vi "daqio_get_dashboard.vi"(8 "error in":errorcluster, 11 "daq.io type in":T3={"daq.io ref"=refnum, "daq.io API Base"="http://dashboard.daq.io/api/v1", "Device Key"="", "Account ID"="", "online"=TRUE, "SSL"=TRUE, "buffer"=TRUE}) -> (0 "error out":errorcluster, 2 "dashboards":T1, 3 "daq.io type out":T3={"daq.io ref"=refnum, "daq.io API Base"="http://dashboard.daq.io/api/v1", "Device Key"="", "Account ID"="", "online"=TRUE, "SSL"=TRUE, "buffer"=TRUE})   [LabVIEW 2013, in "daqio minimal.lvlib"]
doc: "This VI creates a new default dashboard for a specific account and makes it the new default dashboard for the current device."
uses:
  daqio minimal.lvlib
  _typedefs/daqio-Type.ctl
  <vilib>/httpClient/ClientHandle.ctl
  _typedefs/daqio-Device-Just-Dashboards.ctl
  _typedefs/daqio-Device-Dashboards.ctl
  <vilib>/Easy HTTP Client/Easy HTTP.lvlib
  <vilib>/httpClient/LabVIEWHTTPClient.lvlib
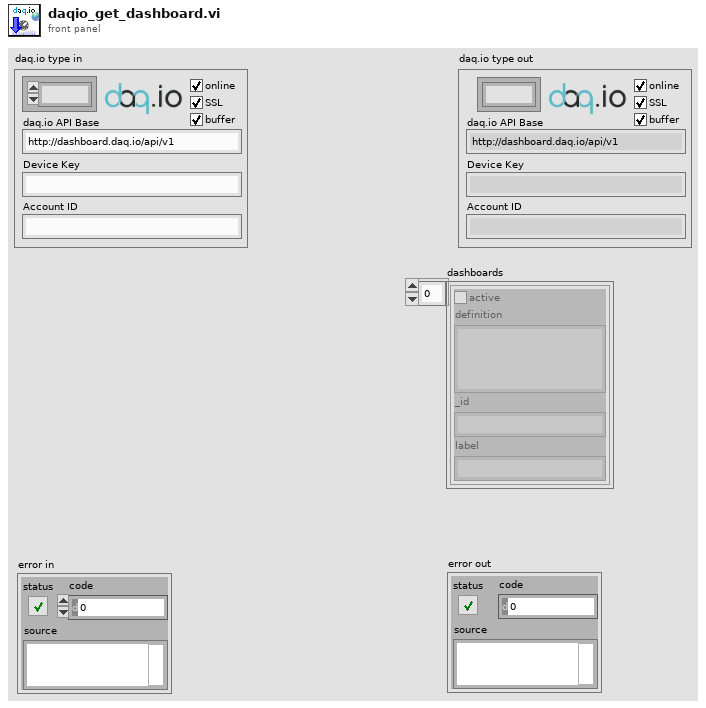
[diagram p1: front panel]
types:
  T1 = typedef "daqio minimal.lvlib/daqio-Device-Just-Dashboards.ctl" = T2[]
  T2 = typedef "daqio minimal.lvlib/daqio-Device-Dashboards.ctl" = cluster{"active":bool, "definition":string, "_id":string, "label":string}
  T3 = typedef "daqio minimal.lvlib/daqio-Type.ctl" = cluster{"daq.io ref":T4, "daq.io API Base":string, "Device Key":string, "Account ID":string, "online":bool, "SSL":bool, "buffer":bool}
  T4 = typedef "LabVIEWHTTPClient.lvlib/ClientHandle.ctl" = refnum<k1>
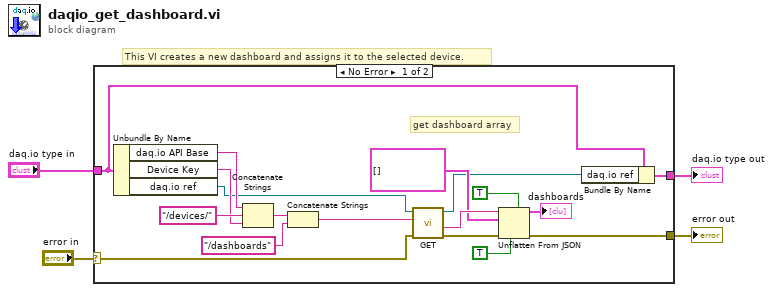
[diagram p0: block diagram]
diagram:
  # "This VI creates a new dashboard and assigns it to the selected device."
  n1 = case shown="No Error" "error in" {
    selector: "error in" -> [w8 w23]
    tunnel: "daq.io type in" -> [w10 w24]
    tunnel: [w21 w24] -> w3
    tunnel: [w5 w23] -> w2
    frame No Error {
      # "get dashboard array"
      n2 = Unbundle By Name(w10) -> ("daq.io API Base"=w20:string, "Device Key"=w18:string, "daq.io ref"=w9:T4)
      n3 = Concatenate Strings(w20, "/devices/" ("string"), w18) -> (w11:string)
      n4 = Concatenate Strings(w11, "/dashboards") -> (w13:string)
      n5 = call <vilib>:"GET.vi"("error in (no error)"=w8, "url"=w13, "client handle"=w9) -> ("error out"=w14:errorcluster, "body"=w17:string, "client handle out"=w7:T4)  [unwired: 4 in, 2 out]
      n6 = Unflatten From JSON(enable LabVIEW extensions? (T)=TRUE, JSON string=w17, type and defaults=T1 [] ("dashboards"), default null elements? (F)=TRUE, error in (no error)=w14) -> (value=→"dashboards":T1, error out=w5:errorcluster)  [unwired: 2 in]
      n7 = Bundle By Name(cluster=w10, "daq.io ref"=w7) -> (w21:T3)
    }
    frame Error {
    }
  }
  "error out" <- w2
  "daq.io type out" <- w3
